vi "Mean_stdev_Calculation.vi"(10 "Coincidences":i32[](array[numeric]), 11 "MH_UIThread_Data in":T1 {"Acquisitions" min=0 max=100000000 step=1; "T2 Coincidence Cluster"."Stdev" format="%0.2f"; "T2 Coincidence Cluster"."Mean" format="%0.2f"; "Mode" items=["HIST"=0, "T2"=2, "T3"=3]; "SyncDeadTime" min=800 max=160000 step=1; "SyncEdge" items=["falling", "rising"]; "SyncDivider" items=["1", "2", "4", "8", "16"]; "SyncOffset" min=0 max=100000 step=1; "SyncLevel" min=0 max=800 step=1; "AcqTime" min=1 max=360000 step=1; "Binning" items=["1", "2", "4", "8", "16", "32", "64", "128", "256", "512", "1024", "2048", "4096", "8192", "16384", "32768", "65536", "131072", "262144", "524288", "1048576", "2097152", "4194304", "8388608", "16777216", "3355443225"]; "HistoOffset" min=0 max=500 step=1; "HistoLen" min=1024 max=65536 step=1024; "Channels"."DeadTime" min=800 max=160000 step=1; "Channels"."Edge" items=["falling", "rising"]; "Channels"."Offset" min=-100000 max=100000 step=10; "Channels"."Level" min=-1200 max=1200 step=1}) -> (2 "MH_UIThread_Data out":T1 {"Acquisitions" min=0 max=100000000 step=1; "T2 Coincidence Cluster"."Stdev" format="%0.2f"; "T2 Coincidence Cluster"."Mean" format="%0.2f"; "Mode" items=["HIST"=0, "T2"=2, "T3"=3]; "SyncDeadTime" min=800 max=160000 step=1; "SyncEdge" items=["falling", "rising"]; "SyncDivider" items=["1", "2", "4", "8", "16"]; "SyncOffset" min=0 max=100000 step=1; "SyncLevel" min=0 max=800 step=1; "AcqTime" min=1 max=360000 step=1; "Binning" items=["1", "2", "4", "8", "16", "32", "64", "128", "256", "512", "1024", "2048", "4096", "8192", "16384", "32768", "65536", "131072", "262144", "524288", "1048576", "2097152", "4194304", "8388608", "16777216", "3355443225"]; "HistoOffset" min=0 max=500 step=1; "HistoLen" min=1024 max=65536 step=1024; "Channels"."DeadTime" min=800 max=160000 step=1; "Channels"."Edge" items=["falling", "rising"]; "Channels"."Offset" min=-100000 max=100000 step=10; "Channels"."Level" min=-1200 max=1200 step=1}, 3 "T2 Coincidences":i32[][](graph))   [LabVIEW 2023]
uses:
  ConcreteClasses/ConcreteInstrumentClasses/Multiharp/Multiharp/Types/MH_UIThread_Data_SPI.ctl
  ConcreteClasses/ConcreteInstrumentClasses/Multiharp/Multiharp/_lib/PQ/MultiHarp/MH_InitInfo.ctl
  ConcreteClasses/ConcreteInstrumentClasses/Multiharp/Multiharp/Types/MH_InputChannel.ctl
  ConcreteClasses/ConcreteInstrumentClasses/Multiharp/Multiharp/Types/MH_SetInpChanData.ctl
  ConcreteClasses/ConcreteInstrumentClasses/Multiharp/Multiharp/Types/MH_SetInpChanCmds.ctl
  ConcreteClasses/ConcreteInstrumentClasses/Multiharp/Multiharp/_lib/PQ/MultiHarp/MH_MeasMode.ctl
  <vilib>/Analysis/NI_AALBase.lvlib
  typedefs/typedefs.lvlib
panel:
  # "Sync"
  # "Histogram"
  # "Sync"
  # "Histogram"
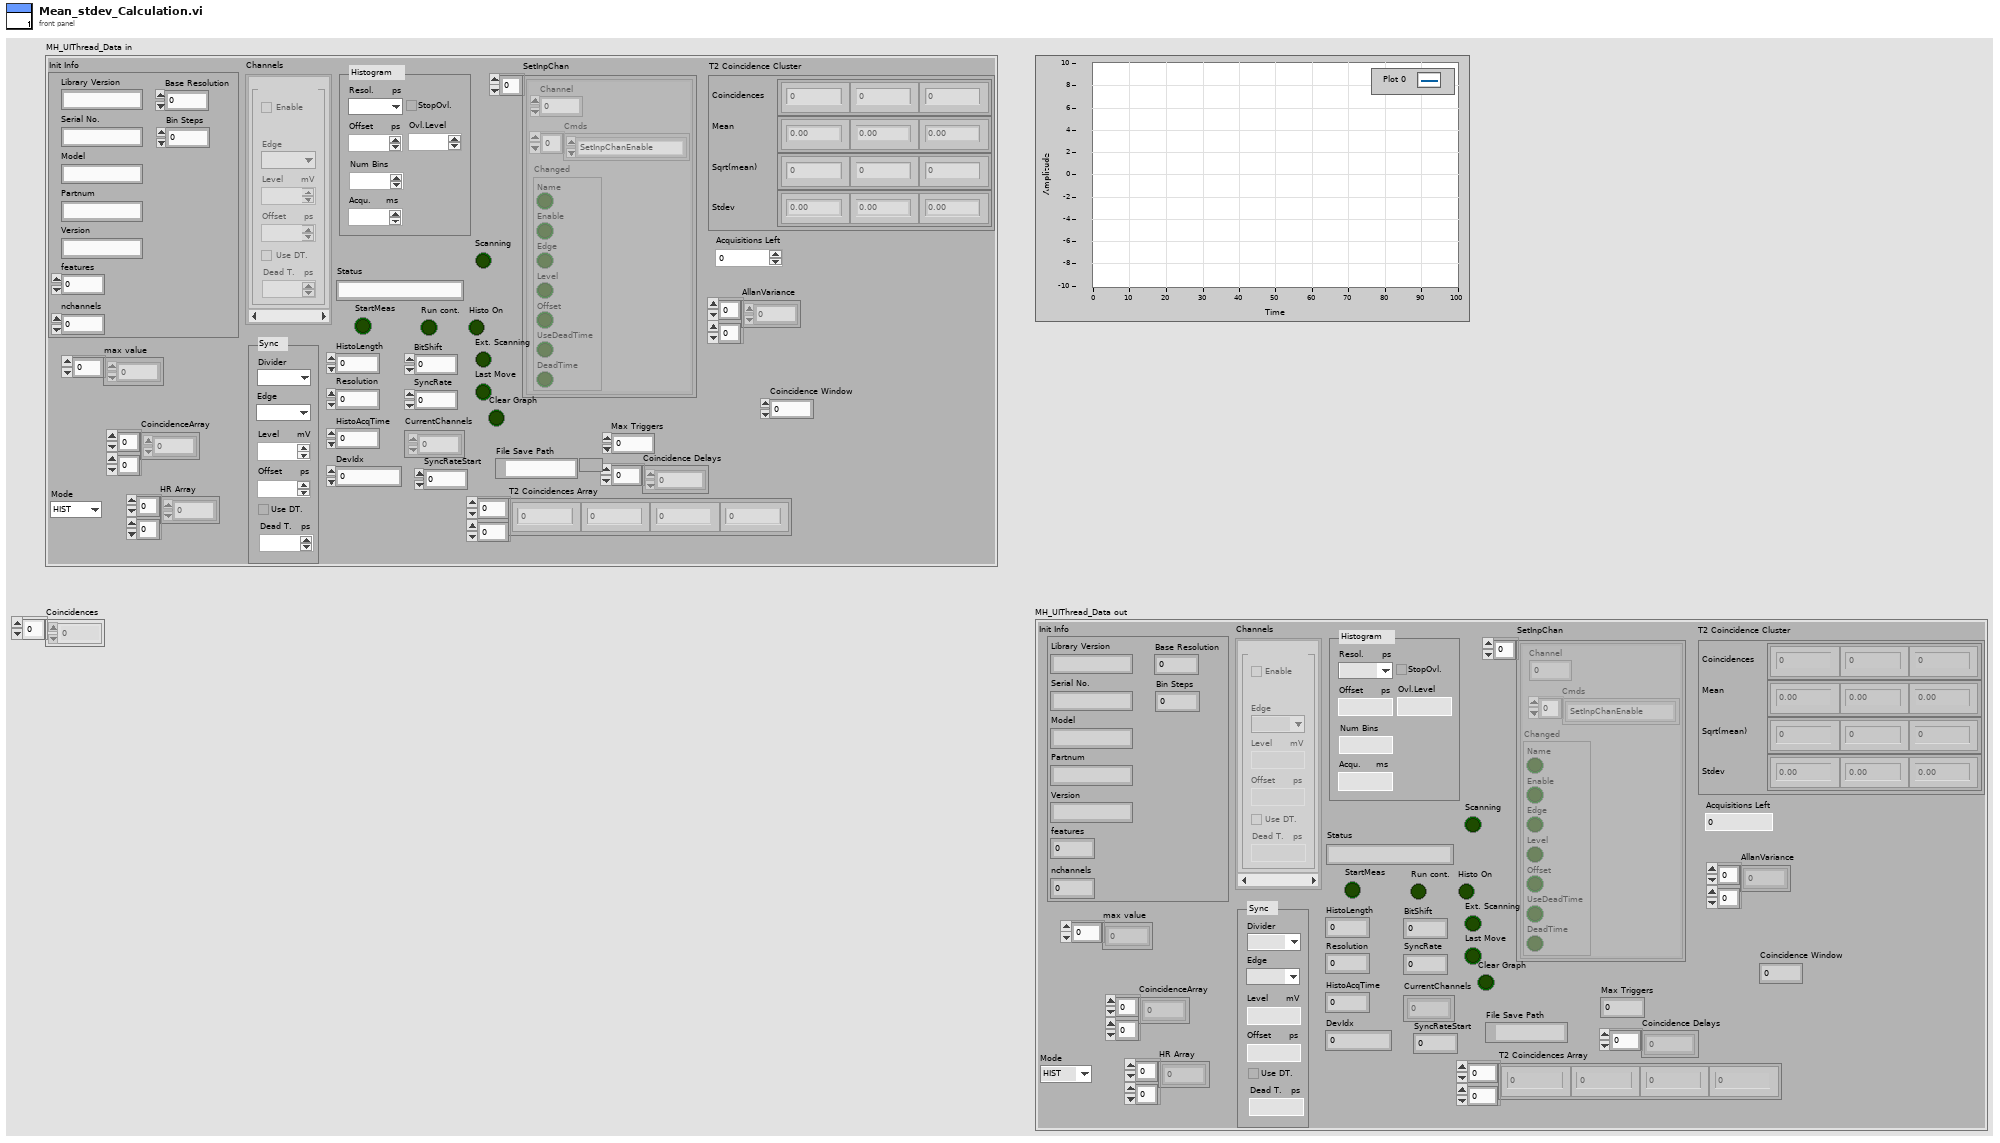
[diagram p1: front panel]
types:
  T1 = typedef "MH_UIThread_Data_SPI.ctl" = cluster{"Init Info":T2, "DevIdx":i32, "SyncDivider":i32, "SyncOffset":i32, "SyncLevel":i32, "Channels":T3[], "CurrentChannels":i32[], "AcqTime":i32, "Binning":i32, "HistoOffset":i32, "HistoLen":i32, "StopOvl.":bool, "OvlLevel":u32, "SyncEdge":i32, "StartMeas":bool, "HistoLength":i32, "Resolution":dbl, "Run cont.":bool, "Status":string, "SyncRate":i32, "BitShift":i32, "HistoAcqTime":dbl, "SyncRateStart":i32, "UseDeadTime":bool, "SyncDeadTime":i32, "SetInpChan":T4[], "max value":u32[], "CoincidenceArray":u32[][], "Histo On":bool, "Mode":T6, "Scanning":bool, "Last Move":bool, "Coincidence Window":dbl, "Max Triggers":i32, "Coincidence Delays":dbl[], "T2 Coincidences Array":i32[][], "Clear Graph":bool, "File Save Path":path, "T2 Coincidence Cluster":cluster{"Coincidences":u32[], "Mean":dbl[], "Sqrt(mean)":dbl[], "Stdev":dbl[]}, "Acquisitions":i32, "HR Array":sgl[][], "Ext. Scanning":bool, "AllanVariance":dbl[][]}
  T2 = typedef "typedefs.lvlib/MH_InitInfo.ctl" = cluster{"Library Version":string, "Serial No.":string, "Model":string, "Partnum":string, "Version":string, "features":i32, "nchannels":i32, "Base Resolution":dbl, "Bin Steps":i32}
  T3 = typedef "MH_InputChannel.ctl" = cluster{"Name":string, "Enable":bool, "Edge":i32, "Level":i32, "Offset":i32, "UseDeadTime":bool, "DeadTime":i32}
  T4 = typedef "MH_SetInpChanData.ctl" = cluster{"Channel":i32, "Cmds":T5[], "Changed":cluster{"Name":bool, "Enable":bool, "Edge":bool, "Level":bool, "Offset":bool, "UseDeadTime":bool, "DeadTime":bool}}
  T5 = typedef "MH_SetInpChanCmds.ctl" = enum16{"SetInpChanEnable", "SetInpChanOffset", "SetInpChanDeadTime", "SetInpChanTrg"}
  T6 = typedef "MH_MeasMode.ctl" = i32
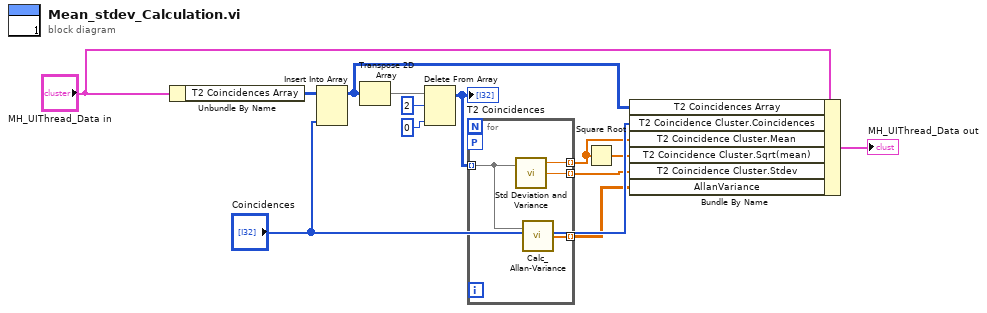
[diagram p0: block diagram]
diagram:
  n1 = Unbundle By Name("MH_UIThread_Data in") -> ("T2 Coincidences Array"=w7:i32[][])
  n2 = Insert Into Array(array=w7, new element="Coincidences") -> (w9:i32[][])  [unwired: 2 in]
  n3 = Transpose 2D Array(2D array=w9) -> (transposed array=w10:i32[][])
  n4 = Delete From Array(array=w10, length=2, index (col)=0 ("index (row)")) -> (array with subset deleted=w13:i32[][])  [unwired: 1 in, 1 out]
  "T2 Coincidences" <- w13
  n5 = for {
    tunnel: w13 -> [w15] mode=indexing
    tunnel: [w17] -> w3 mode=indexing
    tunnel: [w16] -> w2 mode=indexing
    workers-P: _ -> [_]
    tunnel: [w14] -> w1 mode=indexing
    n6 = call <vilib>:"Std Deviation and Variance.vi"("X"=w15) -> ("mean"=w17:dbl, "standard deviation"=w16:dbl)  [unwired: 1 in, 1 out]
    n7 = call "Calc_Allan-Variance.VI"("Input Array"=w15) -> ("AllanVariance"=w14:dbl[])  [unwired: 1 in]
  }
  n8 = Square Root(x=w3) -> (sqrt(x)=w4:dbl[])
  n9 = Bundle By Name(cluster="MH_UIThread_Data in", "T2 Coincidences Array"=w9, "T2 Coincidence Cluster.Coincidences"="Coincidences", "T2 Coincidence Cluster.Mean"=w3, "T2 Coincidence Cluster.Sqrt(mean)"=w4, "T2 Coincidence Cluster.Stdev"=w2, "AllanVariance"=w1) -> (→"MH_UIThread_Data out":T1)
